vi "CheckStatus_Power_HeaterAlarm_.vi"(8 "entrée d'erreur (pas d'erreur)":errorcluster, 9 "DAQmxTask out":refnum<class "DAQmxTask.lvclass">, 10 "RelayKeyStatus":bool, 11 "DAQmxTaskContainer en entrée":refnum<class "DAQmxTaskContainer.lvclass">) -> (0 "sortie d'erreur":errorcluster, 1 "PowerStatus":bool, 2 "PowerStatusChanged":bool, 3 "DAQmxTaskContainer en sortie":refnum<class "DAQmxTaskContainer.lvclass">, 4 "DAQmxTaskAICurrent en sortie":refnum<class "DAQmxTaskAICurrent.lvclass">, 5 "HeaterAlarmStatus":bool, 7 "HeaterAlarmStatusChanged":bool)   [LabVIEW 2015, in "DAQmxTaskContainer.lvclass"]
uses:
  DAQmxTaskContainer/DAQmxTaskContainer.lvclass
  DAQmxTaskAICurrent.lvclass
  DAQmxTaksContainer_General.lvclass
  DAQmxTask.lvclass
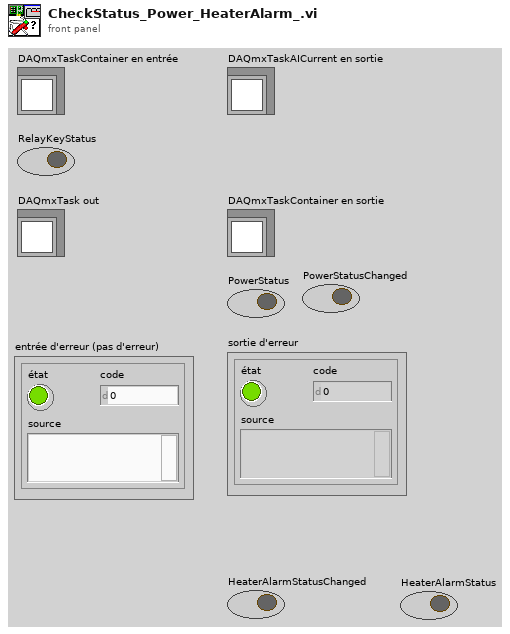
[diagram p1: front panel]
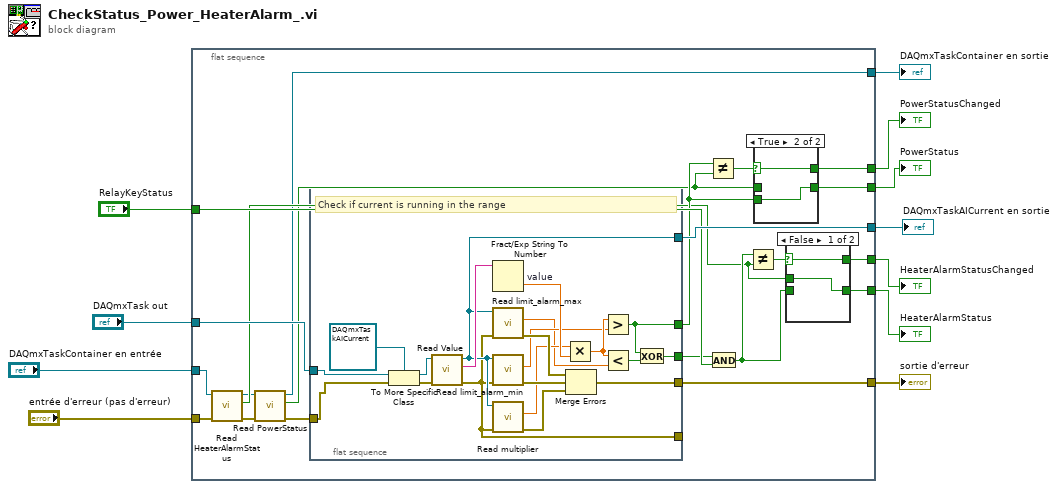
[diagram p0: block diagram]
diagram:
  n1 = flat-sequence {
    tunnel: "DAQmxTask out" -> [w30]
    tunnel: "DAQmxTaskContainer en entrée" -> [w17]
    tunnel: "entrée d'erreur (pas d'erreur)" -> [w14]
    tunnel: [w32] -> w1
    tunnel: [w31] -> w5
    tunnel: "RelayKeyStatus" -> [w29]
    tunnel: [w25] -> w7
    tunnel: [w24] -> w8
    tunnel: [w22] -> w9
    tunnel: [w20] -> w10
    tunnel: [w15] -> w11
    frame #0 {
      n2 = call "Read HeaterAlarmStatus.vi"("error in (no error)"=w14, "DAQmxTaksContainer_General in"=w17) -> ("error out"=w13:errorcluster, "HeaterAlarmStatus"=w19:bool, "DAQmxTaksContainer_General out"=w16:refnum<class "DAQmxTaskContainer.lvclass">)  [unwired: 7 in]
      n3 = call "Read PowerStatus.vi"("error in (no error)"=w13, "DAQmxTaksContainer_General in"=w16) -> ("error out"=w12:errorcluster, "PowerStatus"=w18:bool, "DAQmxTaksContainer_General out"=w15:refnum<class "DAQmxTaskContainer.lvclass">)  [unwired: 7 in]
      n4 = flat-sequence {
        tunnel: [w41] -> w32
        tunnel: [w40] -> w31
        tunnel: [w39] -> _
        tunnel: w30 -> [w36]
        tunnel: [w35] -> w28
        tunnel: [w34] -> w26
        tunnel: w12 -> [w33]
        frame #0 {
          # "Check if current is running in the range"
          n5 = To More Specific Class(target class=refnum<class "DAQmxTaskAICurrent.lvclass"> refnum ("DAQmxTaskAICurrent.lvclass"), reference=w36, error in=w33) -> (specific class reference=w43:refnum<class "DAQmxTaskAICurrent.lvclass">, error out=w42:errorcluster)
          n6 = call-dynamic "Read Value.vi"("error in (no error)"=w42, "DAQmxTaskAICurrent en entrée"=w43) -> ("error out"=w39:errorcluster, "Data string"=w45:string, "DAQmxTaskAICurrent en sortie"=w40:refnum<class "DAQmxTaskAICurrent.lvclass">)  [unwired: 6 in, 1 out]
          n7 = Fract/Exp String To Number "value"(string=w45) -> (number=w50:dbl)  [unwired: 3 in, 1 out]
          n8 = call "Read limit_alarm_max.vi"("error in (no error)"=w39, "DAQmxTaskAICurrent en entrée"=w40) -> ("error out"=w47:errorcluster, "limit_alarm_max"=w37:dbl)  [unwired: 7 in, 1 out]
          n9 = call "Read limit_alarm_min.vi"("error in (no error)"=w39, "DAQmxTaskAICurrent en entrée"=w40) -> ("error out"=w48:errorcluster, "limit_alarm_min"=w38:dbl)  [unwired: 7 in, 1 out]
          n10 = call "Read multiplier.vi"("error in (no error)"=w39, "DAQmxTaskAICurrent en entrée"=w40) -> ("error out"=w49:errorcluster, "multiplier"=w46:dbl)  [unwired: 7 in, 1 out]
          n11 = Multiply(x=w46, y=w50) -> (x*y=w51:dbl)
          n12 = Merge Errors(w47, w48, w49) -> (w41:errorcluster)
          n13 = Greater?(x=w51, y=w38) -> (0:w34:bool)
          n14 = Less?(x=w51, y=w37) -> (x < y?=w52:bool)
          n15 = Exclusive Or(1:w52, 2:w34) -> (0:w35:bool)
        }
      }
      n16 = Not Equal?(x=w26, y=w18) -> (x != y?=w27:bool)
      n17 = And(x=w28, y=w29) -> (x .and. y?=w21:bool)
      n18 = Not Equal?(x=w21, y=w19) -> (x != y?=w23:bool)
      n19 = case shown="True" w27 {
        selector: w27 -> [w58 w59]
        tunnel: [w58 w59] -> w25
        tunnel: w26 -> [_ w60]
        tunnel: [w57 w60] -> w24
        tunnel: w18 -> [w57 _]
        frame False {
        }
        frame True {
        }
      }
      n20 = case shown="False" w23 {
        selector: w23 -> [w54 w56]
        tunnel: [w54 w56] -> w22
        tunnel: [w53 w55] -> w20
        tunnel: w21 -> [_ w55]
        tunnel: w19 -> [w53 _]
        frame False {
        }
        frame True {
        }
      }
    }
  }
  "DAQmxTaskContainer en sortie" <- w11
  "HeaterAlarmStatus" <- w10
  "HeaterAlarmStatusChanged" <- w9
  "PowerStatus" <- w8
  "PowerStatusChanged" <- w7
  "sortie d'erreur" <- w1
  "DAQmxTaskAICurrent en sortie" <- w5
